vi "Previous VI.vi"(0 "PDF Report IN":T21(xcontrol), 11 "error in (no error)":errorcluster) -> (4 "PDF Report OUT":T21(xcontrol), 8 "Execute Actual VI":bool, 15 "error out":errorcluster)   [LabVIEW 2012]
doc: "Version 1.0\nDeveloped by Jean-Marc Simard\nCopyright © 2010, Exaprom Inc.\nAll rights reserved.\nLicense: BSD\n\nWith iTextSharp 4.1.6 (http://itextsharp.sourceforge.net)\nunder Mozilla Public License Version 1.1\n(http://www.mozilla.org/MPL/MPL-1.1.html)"
uses:
  Controls/PDF Report Xcontrol/PDF Report.xctl
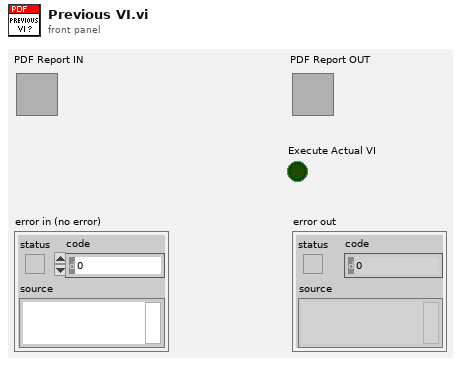
[diagram p1: front panel]
types:
  T1 = typedef "Font cluster.ctl" = cluster{"Name":string, "Size":T2, "Color":T3, "Style":cluster{"Bold":bool, "Italic":bool, "Underline":bool, "Strikeout":bool}}
  T2 = typedef "Font size.ctl" = sgl
  T3 = typedef "Font color.ctl" = u32
  T4 = typedef "Unit.ctl" = enum16{"inch", "mm"}
  T5 = typedef "Paragraphe cluster.ctl" = cluster{" Aligment":T6, "Line spacing":T7}
  T6 = typedef "Texte alignement.ctl" = enum16{"Select", "CENTER", "JUSTIFY", "LEFT", "RIGHT"}
  T7 = typedef "Line spacing.ctl" = enum16{"Select", "1.0", "1.5", "2.0"}
  T8 = typedef "Page dimensions.ctl" = cluster{"Start at page":i32, "Orientation":T9, "widht":sgl, "height":sgl, "Margin left":sgl, "Margin right":sgl, "Margin top":sgl, "Margin bottom":sgl}
  T9 = typedef "Page Orientation.ctl" = enum16{"Portrait", "Landscape"}
  T10 = typedef "Image or Table Caption.ctl" = cluster{"Caption":string, "Separator":string, "Position":enum16{"Above", "Below"}}
  T11 = typedef "Header Footer [ ].ctl" = T12[]
  T12 = typedef "Header Footer cluster.ctl" = cluster{"Start page":i32, "Type":T13, "Alignment":T14, "Vertical Alignement":T15, "Image (%)":sgl, "Page #":T16, "Text":string, "Path":string, "Font":T1, "Font refnum":refnum<k24>, "Line":cluster{"Line":T17, "Thickness (points)":sgl, "Colour":T3}}
  T13 = typedef "Header Footer Type.ctl" = enum16{"Select", "Text", "Text + hyperlink", "Page number", "Image", "Image + hyperlink"}
  T14 = typedef "Header footer horiz alignment.ctl" = enum16{"Left", "Center", "Right"}
  T15 = typedef "Cell Vertical alignment.ctl" = enum16{"TOP", "MIDDLE", "BOTTOM"}
  T16 = typedef "Page number.ctl" = cluster{"Text 1":string, "Text 2":string, "Text 3":string}
  T17 = typedef "Header Footer Line.ctl" = enum16{"No line", "Horizontal line"}
  T18 = typedef "Watermark cluster2.ctl" = cluster{"Show? (F)":bool, "Type":enum16{"Image", "Text"}, "Opacity (%)":sgl, "Rotate(°)":sgl, "Position":cluster{"Position":T19, "X":sgl, "Y":sgl}, "Image path":path, "Scaled(%)":sgl, "Image refnum":refnum<k24>, "Text":string, "Font":cluster{"Name":string, "Size":T2, "Color":T3}, "Font refnum":refnum<k24>, "Alignment":T14, "Automatic":bool}
  T19 = typedef "Watermark Position.ctl" = enum16{"Absolute", "Center (page)", "Center (text section)"}
  T20 = typedef "System Fonts.ctl" = cluster{"Font name [ ]":string[], "Font and file names [ ]":cluster{"Font name":string, "File name":string}[]}
  T21 = cluster{"Document":refnum<k24>, "Writer":refnum<k24>, "Default Font":refnum<k24>, "Default Font cluster":T1, "Path":path, "Unit (default = mm)":T4, "Paragraphe cluster":T5, "Pages dimensions [ ]":T8[], "Captions":cluster{"Image":T10, "Image counter":u16, "Table":T10, "Table counter":u16, "Font":T1}, "Header":T11, "Footer":T11, "Watermark ":T18, "Actual VI name":string, "System Fonts":T20}
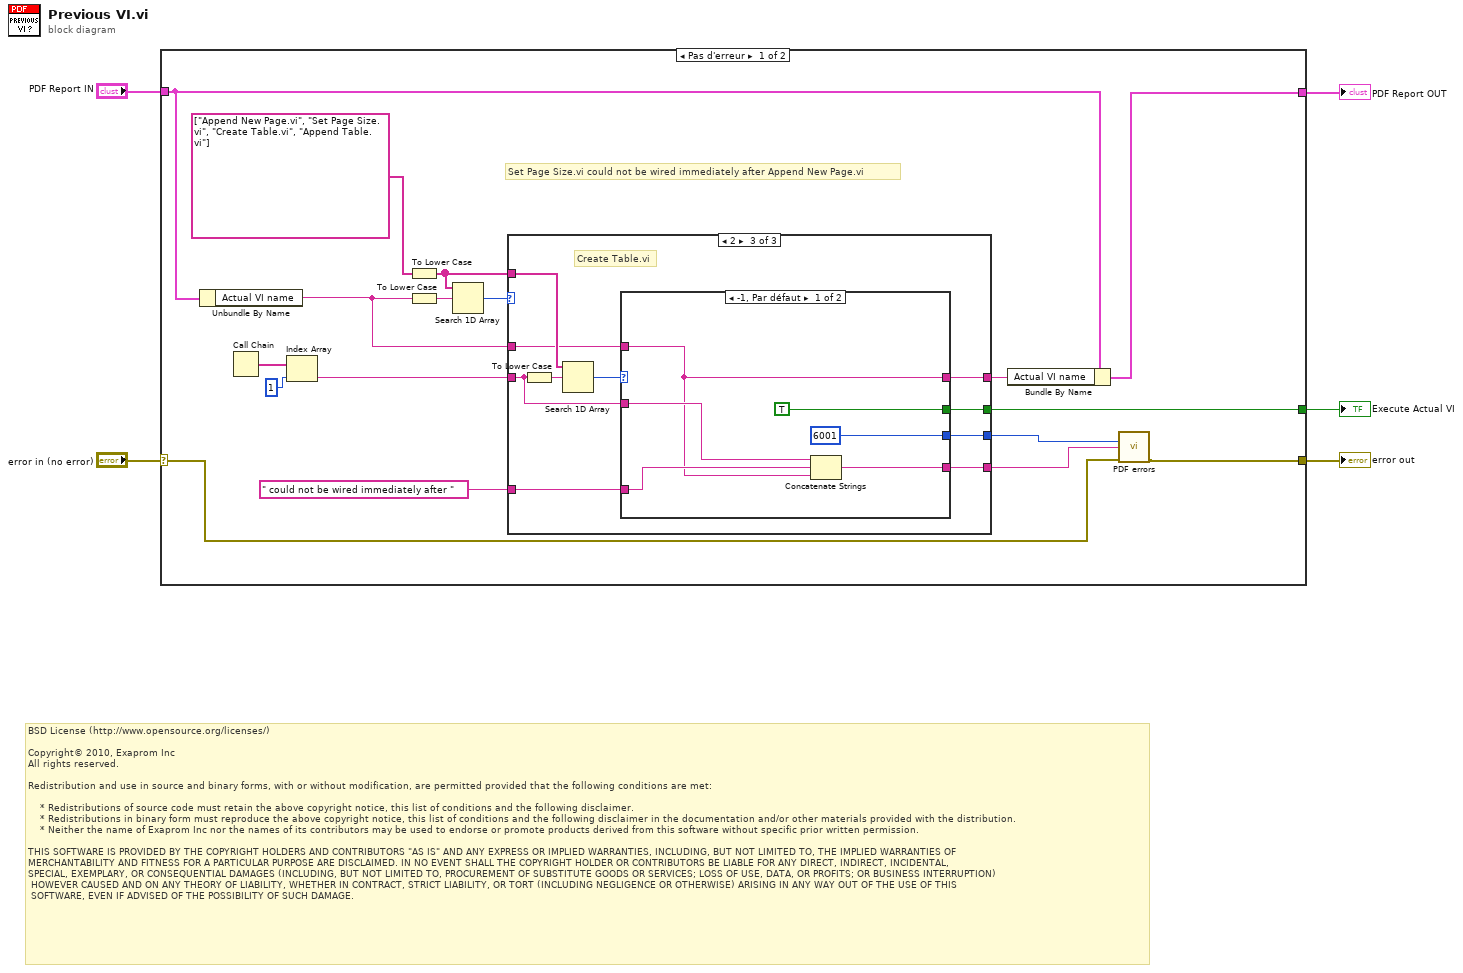
[diagram p0: block diagram]
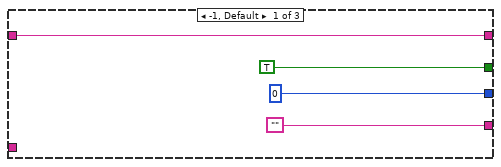
[diagram p2: hidden frame]
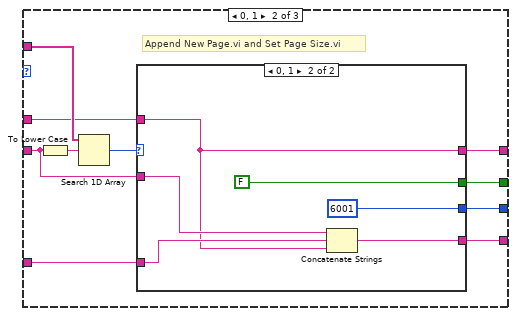
[diagram p3: hidden frame]
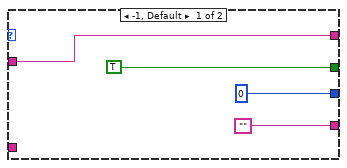
[diagram p4: hidden frame]
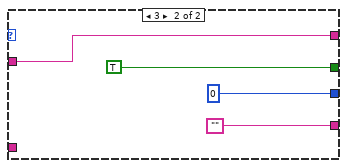
[diagram p5: hidden frame]
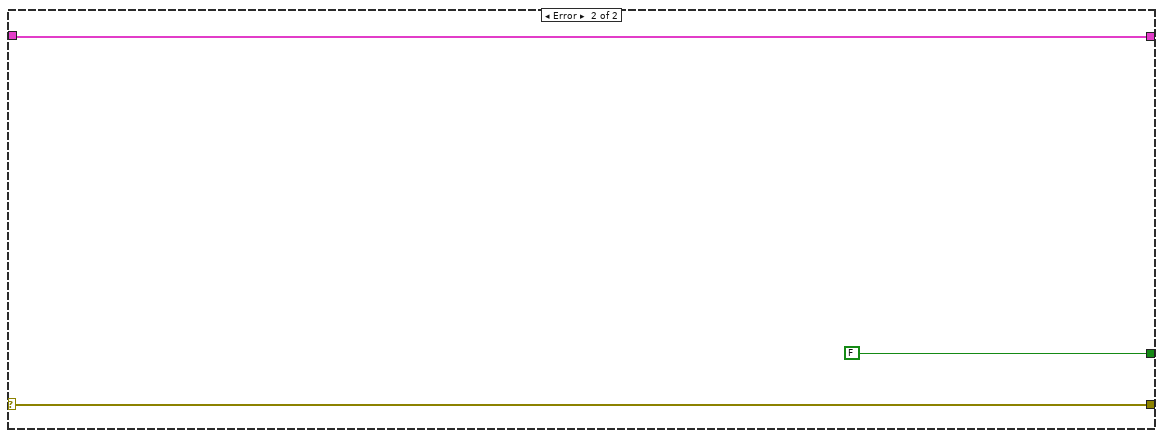
[diagram p6: hidden frame]
diagram:
  # "BSD License (http://www.opensource.org/licenses/)\n\nCopyright© 2010, Exaprom Inc\nAll rights reserved.\n\nRedistribution and use in source and binary forms, with or without modification, are permitted provided that the following conditions are met:\n\n    * Redistributions of source code must retain the above copyright notice, this list of conditions and the following disclaimer.\n    * Redistributions in binary form must reproduce the above copyright notice, this list of conditions and the following disclaimer in the documentation and/or other materials provided with the distribution.\n    * Neither the name of Exaprom Inc nor the names of its contributors may be used to endorse or promote products derived from this software without specific prior written permission.\n\nTHIS SOFTWARE IS PROVIDED BY THE COPYRIGHT HOLDERS AND CONTRIBUTORS \"AS IS\" AND ANY EXPRESS OR IMPLIED WARRANTIES, INCLUDING, BUT NOT LIMITED TO, THE IMPLIED WARRANTIES OF \nMERCHANTABILITY AND FITNESS FOR A PARTICULAR PURPOSE ARE DISCLAIMED. IN NO EVENT SHALL THE COPYRIGHT HOLDER OR CONTRIBUTORS BE LIABLE FOR ANY DIRECT, INDIRECT, INCIDENTAL,\nSPECIAL, EXEMPLARY, OR CONSEQUENTIAL DAMAGES (INCLUDING, BUT NOT LIMITED TO, PROCUREMENT OF SUBSTITUTE GOODS OR SERVICES; LOSS OF USE, DATA, OR PROFITS; OR BUSINESS INTERRUPTION)\n HOWEVER CAUSED AND ON ANY THEORY OF LIABILITY, WHETHER IN CONTRACT, STRICT LIABILITY, OR TORT (INCLUDING NEGLIGENCE OR OTHERWISE) ARISING IN ANY WAY OUT OF THE USE OF THIS\n SOFTWARE, EVEN IF ADVISED OF THE POSSIBILITY OF SUCH DAMAGE."
  n1 = case shown="Pas d'erreur" "error in (no error)" {
    selector: "error in (no error)" -> [w9 w69]
    tunnel: "PDF Report IN" -> [w18 w68]
    tunnel: [w17 w68] -> w4
    tunnel: [w6 w69] -> w3
    tunnel: [w7 FALSE] -> w1
    frame No Error {
      # "Set Page Size.vi could not be wired immediately after Append New Page.vi"
      n2 = Unbundle By Name(w18) -> ("Actual VI name"=w12:string)
      n3 = Call Chain() -> (call chain=w20:string[])
      n4 = Index Array(array=w20, index=1) -> (element=w11:string)
      n5 = To Lower Case(string=string[] ["Append New Page.vi", "Set Page Size.vi", "Create Table.vi", "Append Table.vi"]) -> (all lower case string=w14:string[])
      n6 = To Lower Case(string=w12) -> (all lower case string=w21:string)
      n7 = Search 1D Array(1D array=w14, element=w21) -> (index of element=w13:i32)  [unwired: 1 out]
      n8 = case shown="2" w13 {
        tunnel: w11 -> [w26 w32 w52]
        tunnel: w12 -> [_ w31 w51]
        tunnel: [w26 w33 w53] -> w8
        tunnel: w14 -> [_ w35 w55]
        tunnel: [TRUE w30 w50] -> w7
        tunnel: " could not be wired immediately after " -> [_ w29 w49]
        tunnel: ["" w28 w47] -> w16
        tunnel: [0 ("y") w27 w48] -> w15
        frame -1, Default {
        }
        frame 0, 1 {
          # "Append New Page.vi and Set Page Size.vi"
          n9 = To Lower Case(string=w32) -> (all lower case string=w36:string)
          n10 = Search 1D Array(1D array=w35, element=w36) -> (index of element=w34:i32)  [unwired: 1 out]
          n11 = case shown="0, 1" w34 {
            tunnel: [w40 w43] -> w33
            tunnel: w32 -> [w40 w44]
            tunnel: w31 -> [_ w43]
            tunnel: [TRUE FALSE] -> w30
            tunnel: w29 -> [_ w45]
            tunnel: ["" w42] -> w28
            tunnel: [0 ("y") 6001 ("y")] -> w27
            frame -1, Default {
            }
            frame 0, 1 {
              n12 = Concatenate Strings(w44, w45, w43) -> (w42:string)
            }
          }
        }
        frame 2 {
          # "Create Table.vi"
          n13 = To Lower Case(string=w52) -> (all lower case string=w56:string)
          n14 = Search 1D Array(1D array=w55, element=w56) -> (index of element=w54:i32)  [unwired: 1 out]
          n15 = case shown="-1, Par défaut" w54 {
            tunnel: [w59 w65] -> w53
            tunnel: w52 -> [w60 w65]
            tunnel: w51 -> [w59 _]
            tunnel: [TRUE TRUE] -> w50
            tunnel: w49 -> [w61 _]
            tunnel: [6001 ("y") 0 ("y")] -> w48
            tunnel: [w58 ""] -> w47
            frame -1, Default {
              n16 = Concatenate Strings(w60, w61, w59) -> (w58:string)
            }
            frame 3 {
            }
          }
        }
      }
      n17 = Bundle By Name(cluster=w18, "Actual VI name"=w8) -> (w17:T21)
      n18 = call "PDF errors.vi"("code"=w15, "Additionnal information"=w16, "error in (no error)"=w9) -> ("error out"=w6:errorcluster)  [unwired: 12 out]
    }
    frame Error {
    }
  }
  "PDF Report OUT" <- w4
  "error out" <- w3
  "Execute Actual VI" <- w1
